vi "pr1a2.vi"() -> ()   [LabVIEW 2013]
uses:
  <vilib>/Utility/error.llb/DialogType.ctl
  <vilib>/DAQmx/write.llb/DAQmx Write (Analog Wfm 1Chan NSamp).vi
  <vilib>/DAQmx/create/channels.llb/DAQmx Create Channel (AO-Voltage-Basic).vi
  <vilib>/DAQmx/configure/timing.llb/DAQmx Timing (Use Waveform).vi
  <vilib>/DAQmx/miscellaneous.llb/DAQmx Fill In Error Info.vi
  <vilib>/measure/NI_MABase.lvlib
panel:
  out "signal out":waveform(dbl)
  in  "Canal generar":tag
  in  "Valor maximo generar":dbl=10.0 format="%0.2f"
  in  "Valor minimo generar":dbl=-10.0 format="%0.2f"
  in  "sampling info":cluster{"Fs":dbl, "#s":dbl}={"Fs"=1000.0, "#s"=1000.0} {"Fs" format="%.2p"}
  in  "amplitude":dbl=1.0 format="%0.2p"
  in  "frequency":dbl=10.0 format="%0.2p"
  out "Waveform Chart":waveform(dbl)(graph)
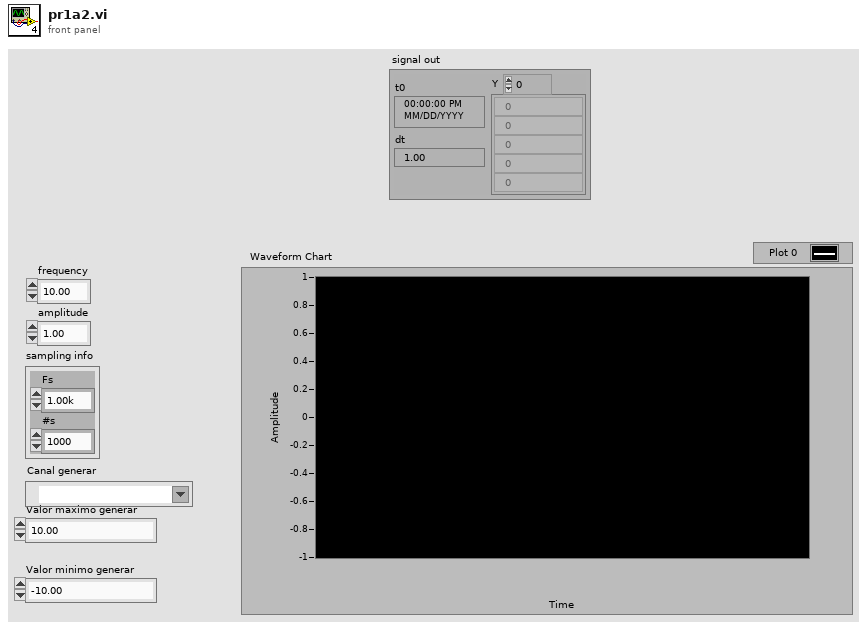
[diagram p1: front panel]
types:
  T1 = typedef "DialogType.ctl" = u16
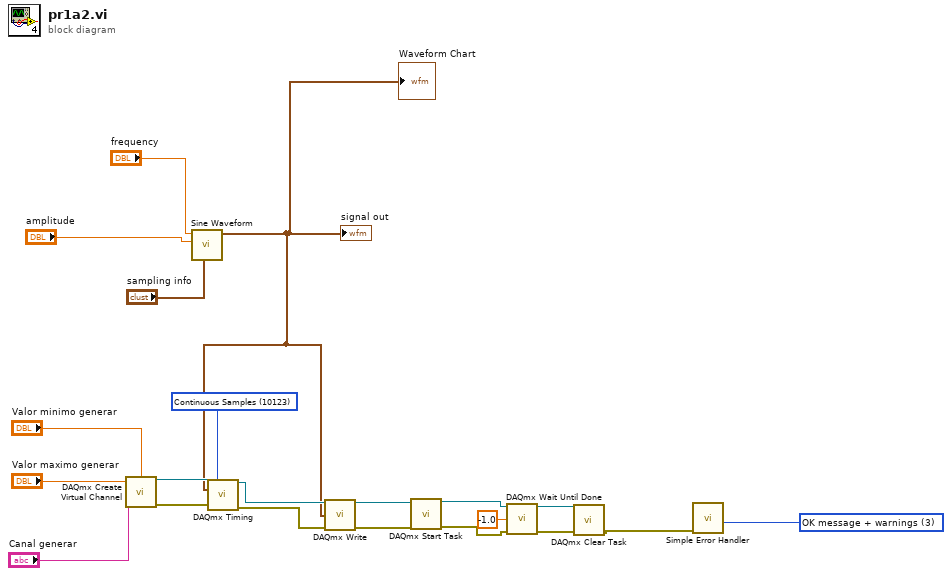
[diagram p0: block diagram]
diagram:
  w5 = T1 3 items=["no dialog", "OK message", "continue or stop message", "OK message + warnings", "continue/stop + warnings"] ("type of dialog (OK msg:1)")
  w15 = 10123 items=["Finite Samples"=10178, "Continuous Samples"=10123, "Hardware Timed Single Point"=12522] ("sample mode")
  n1 = call-poly <vilib>:"DAQmx Create Virtual Channel.vi"("maximum value"="Valor maximo generar", "minimum value"="Valor minimo generar", "physical channels"="Canal generar") -> ("task out"=w20:refnum<k21>, "error out"=w14:errorcluster)  [unwired: 11 in]
  n2 = call <vilib>:"Sine Waveform.vi"("sampling info"="sampling info", "amplitude"="amplitude", "frequency"="frequency") -> ("signal out"=w3:waveform(dbl))  [unwired: 7 in, 1 out]
  "Waveform Chart" <- w3
  "signal out" <- w3
  n3 = call-poly <vilib>:"DAQmx Timing.vi"("task/channels in"=w20, "sample mode"=w15, "waveform"=w3, "error in"=w14) -> ("task out"=w19:refnum<k21>, "error out"=w13:errorcluster)  [unwired: 10 in]
  n4 = call-poly <vilib>:"DAQmx Write.vi"("task/channels in"=w19, "data"=w3, "error in"=w13) -> ("task out"=w18:refnum<k21>, "error out"=w12:errorcluster)  [unwired: 10 in, 1 out]
  n5 = call <vilib>:"DAQmx Start Task.vi"("task/channels in"=w18, "error in"=w12) -> ("task out"=w17:refnum<k21>, "error out"=w11:errorcluster)  [unwired: 12 in]
  n6 = call <vilib>:"DAQmx Wait Until Done.vi"("task/channels in"=w17, "timeout (sec)"=-1.0, "error in"=w11) -> ("task out"=w16:refnum<k21>, "error out"=w10:errorcluster)  [unwired: 11 in]
  n7 = call <vilib>:"DAQmx Clear Task.vi"("task in"=w16, "error in"=w10) -> ("error out"=w4:errorcluster)  [unwired: 13 in]
  n8 = call <vilib>:"Simple Error Handler.vi"("type of dialog (OK msg:1)"=w5, "error in (no error)"=w4) -> ()  [unwired: 3 in, 5 out]
